vi "get piece from cube  3.vi"() -> ()   [LabVIEW 2018]
uses:
  vision/vision info 2.vi
panel:
  in  "x":dbl
  in  "z1 2":dbl
  in  "z2 2":dbl
  in  "step 2":dbl
  in  "speed 2":i32
  in  "move arm":bool
  out "_y":dbl
  out "_x":dbl
  in  "take2":bool
  in  "grip":bool
  in  "base":i32(slide) scale=-125.0..125.0
  in  "c1":i8
  in  "c2":i8
  in  "camera mode":bool
  in  "z1":dbl
  in  "z2":dbl
  in  "step":dbl
  in  "speed 1":i32
  in  "y_plus":dbl
  in  "take":bool
  in  "x_plus":dbl
  in  "move":bool
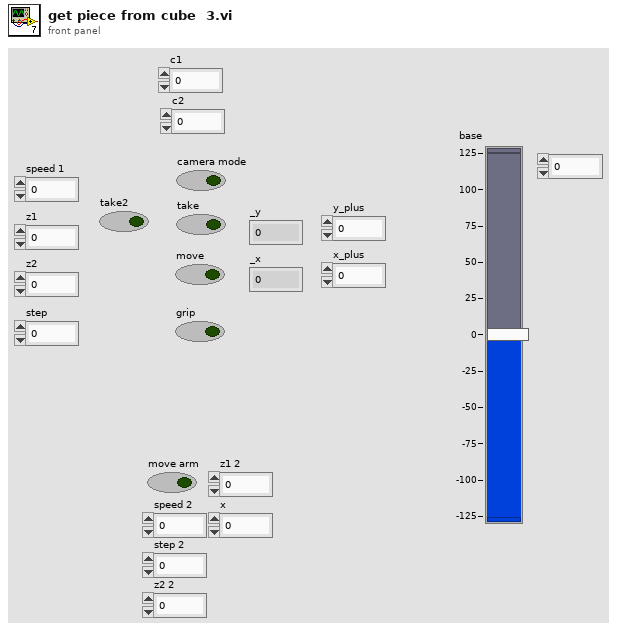
[diagram p1: front panel]
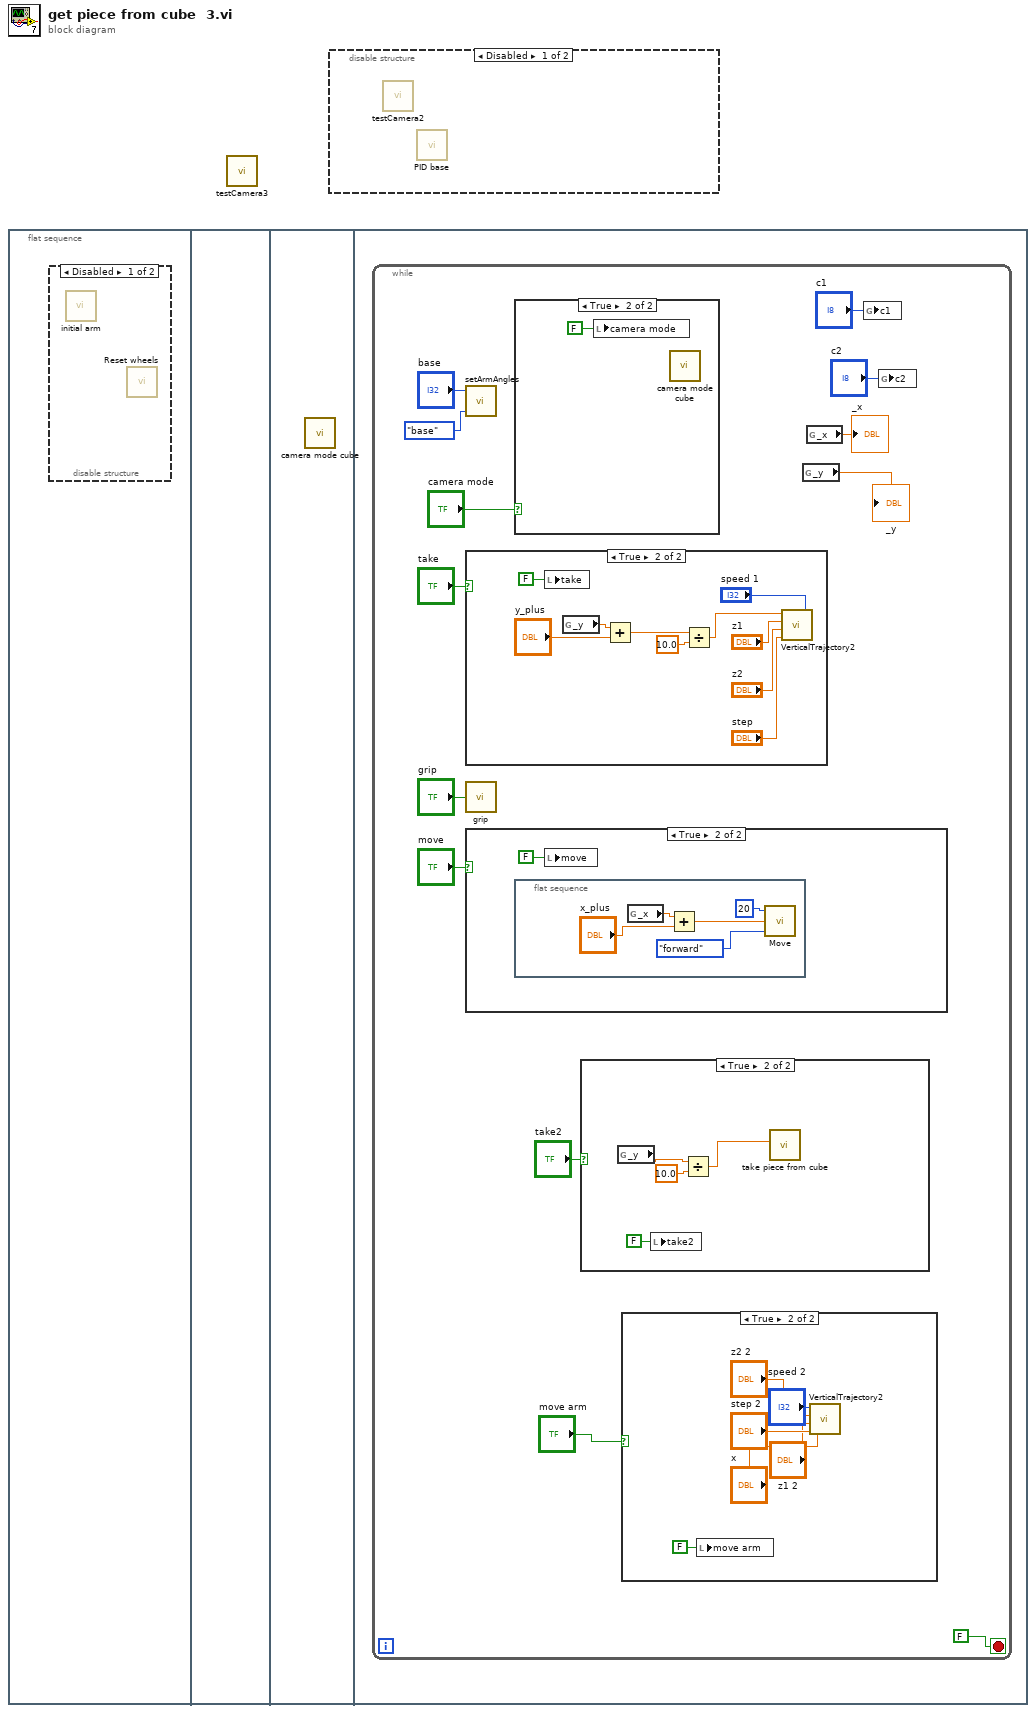
[diagram p0: block diagram]
diagram:
  n1 = flat-sequence {
    frame #0 {
      n2 = disable-structure shown="Disabled" {
        frame Disabled {
          n3 = call "initial arm.vi"() -> ()  [unwired: 12 in]
          n4 = call "Reset wheels.vi"() -> ()  [unwired: 12 in]
        }
        frame Enabled {
        }
      }
    }
    frame #1 {
    }
    frame #2 {
      n5 = call "camera mode cube.vi"() -> ()  [unwired: 12 in]
    }
    frame #3 {
      n6 = while {
        stop <- FALSE stop-if-true
        n7 = call "setArmAngles.vi"("Enum"=enum16{"shoulder", "elbow", "wrist", "base"}."base", "angle"="base") -> ()  [unwired: 2 in]
        n8 = case shown="True" "take" {
          frame False {
          }
          frame True {
            n9 = local write "take"(FALSE ("take")) -> ()
            n10 = global read "vision info 2.vi" "_y"() -> (w34:dbl)
            n11 = Add(x=w34, y="y_plus") -> (x+y=w32:dbl)
            n12 = Divide(x=w32, y=10.0) -> (x/y=w30:dbl)
            n13 = call "VerticalTrajectory2.vi"("speed 1"="speed 1", "step"="step", "z2"="z2", "z1"="z1", "x"=w30) -> ()  [unwired: 3 in]
          }
        }
        n14 = call "grip.vi"("grip"="grip") -> ()
        n15 = case shown="True" "move" {
          frame False {
          }
          frame True {
            n16 = flat-sequence {
              frame #0 {
                n17 = global read "vision info 2.vi" "_x"() -> (w27:dbl)
                n18 = Add(x=w27, y="x_plus") -> (x+y=w25:dbl)
                n19 = call "Move.vi"("Enum"=enum16{"forward", "backward", "left", "right"}."forward", "distance"=w25, "speed"=20) -> ()  [unwired: 1 in]
              }
            }
            n20 = local write "move"(FALSE ("move")) -> ()
          }
        }
        n21 = case shown="True" "camera mode" {
          frame False {
          }
          frame True {
            n22 = local write "camera mode"(FALSE ("camera mode")) -> ()
            n23 = call "camera mode cube.vi"() -> ()  [unwired: 12 in]
          }
        }
        n24 = case shown="True" "take2" {
          frame False {
          }
          frame True {
            n25 = global read "vision info 2.vi" "_y"() -> (w21:dbl)
            n26 = local write "take2"(FALSE ("take2")) -> ()
            n27 = Divide(x=w21, y=10.0) -> (x/y=w20:dbl)
            n28 = call "take piece from cube.vi"("y"=w20) -> ()  [unwired: 10 in]
          }
        }
        n29 = case shown="True" "move arm" {
          frame False {
          }
          frame True {
            n30 = local write "move arm"(FALSE ("move arm")) -> ()
            n31 = call "VerticalTrajectory2.vi"("speed 1"="speed 2", "step"="step 2", "z2"="z2 2", "z1"="z1 2", "x"="x") -> ()  [unwired: 3 in]
          }
        }
        n32 = global read "vision info 2.vi" "_y"() -> (→"_y":dbl)
        n33 = global read "vision info 2.vi" "_x"() -> (→"_x":dbl)
        n34 = global write "vision info 2.vi" "c1"("c1") -> ()
        n35 = global write "vision info 2.vi" "c2"("c2") -> ()
      }
    }
  }
  n36 = call "testCamera3.vi"() -> ()  [unwired: 12 in]
  n37 = disable-structure shown="Disabled" {
    frame Disabled {
      n38 = call "testCamera2.vi"() -> ()  [unwired: 12 in]
      n39 = call "PID base.vi"() -> ()  [unwired: 12 in]
    }
    frame Enabled {
    }
  }
